vi "DI Phase Plot Time Axis.vi"(11 "Array Size":i32) -> (3 "Array":dbl[](array[numeric]))   [LabVIEW 2015]
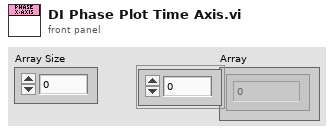
[diagram p1: front panel]
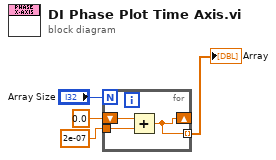
[diagram p0: block diagram]
diagram:
  n1 = for {
    N: "Array Size" -> [_]
    shift-right: [w5] -> _
    shift-left: 0.0 -> [w7]
    tunnel: 2e-07 -> [w6]
    tunnel: [w5] -> w2 mode=indexing
    n2 = Add(x=w7, y=w6) -> (x+y=w5:dbl)
  }
  "Array" <- w2
